vi "Returning Values By Reference Array Of Integers.vi"(7 "newLength":i32, 8 "error in (no error)":errorcluster, 9 "newArray":i32, 10 "length":i32, 11 "x":i32[](array[numeric])=array[4097 elements]) -> (0 "error out":errorcluster, 1 "newArray out":i32, 3 "x out":i32[](array[numeric]), 5 "newLength out":i32)   [LabVIEW 2009, in "LabVIEWWrapper_PassingDataSampleDLL.lvlib"]
doc: "void ReturningValuesByReference_ArrayOfIntegers (int *x, int length, int **newArray, int *newLength);"
uses:
  LabVIEWWrapper_PassingDataSampleDLL.lvlib
  PassingDataSampleDLL.dll
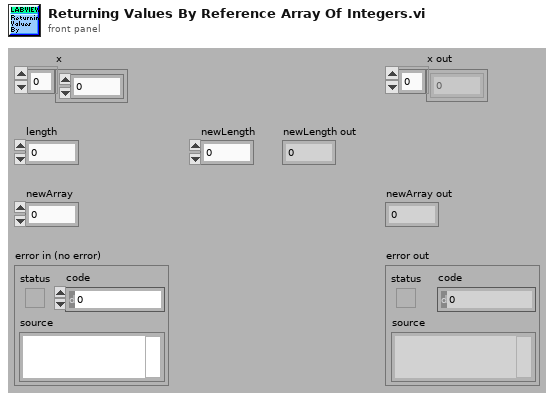
[diagram p1: front panel]
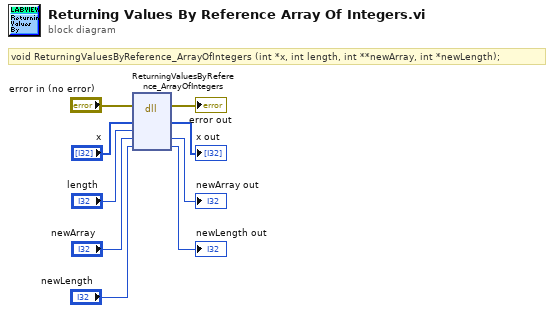
[diagram p0: block diagram]
diagram:
  # "void ReturningValuesByReference_ArrayOfIntegers (int *x, int length, int **newArray, int *newLength);"
  n1 = dll-call lib="C:/My Dropbox/Systems Engineering Application/SDK/C Integration/LabVIEWWrapper/PassingDataSampleDLL.*" fn="ReturningValuesByReference_ArrayOfIntegers"(error in="error in (no error)", "x"="x", "length"="length", "newArray"="newArray", "newLength"="newLength") -> (error out=→"error out":errorcluster, "x"=→"x out":i32[], "newArray"=→"newArray out":i32, "newLength"=→"newLength out":i32)  [unwired: 4 in, 1 out]
